vi "__Local List Menu Delete Handler.vi"(7 "FileManager Data":T1, 8 "error in (no error)":errorcluster) -> (0 "error out":errorcluster)   [LabVIEW 2011]
doc: "Handles the delete operation on the Local list."
uses:
  __File manager Data type.ctl
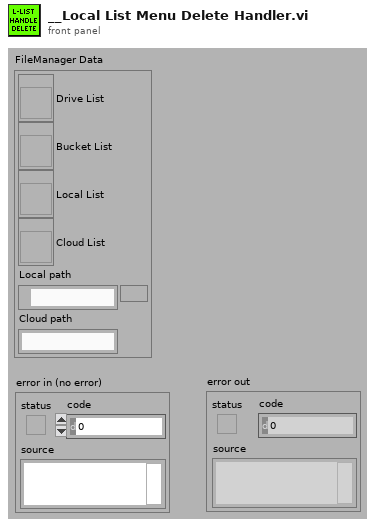
[diagram p1: front panel]
types:
  T1 = typedef "__File manager Data type.ctl" = cluster{"Drive List":refnum<vi>, "Bucket List":refnum<vi>, "Local List":refnum<vi>, "Cloud List":refnum<vi>, "Local path":path, "Cloud path":string}
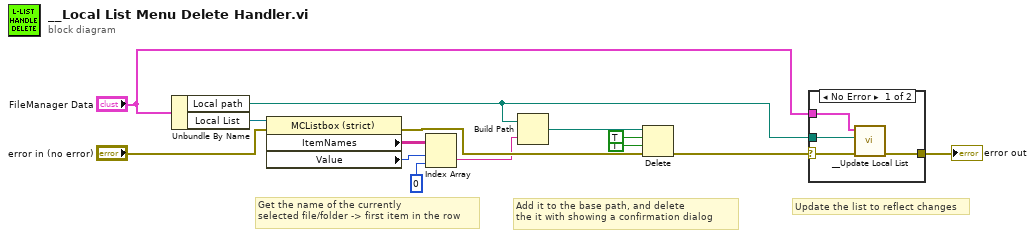
[diagram p0: block diagram]
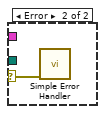
[diagram p2: hidden frame]
diagram:
  # "Update the list to reflect changes"
  # "Add it to the base path, and delete\nthe it with showing a confirmation dialog"
  # "Get the name of the currently\nselected file/folder -> first item in the row"
  n1 = Unbundle By Name("FileManager Data") -> ("Local path"=w3:path, "Local List"=w6:refnum<vi>)
  n2 = property class="MCListbox (strict)"(reference=w6, error in="error in (no error)") -> (error out=w4:errorcluster, "ItemNames"=w9:string[][], "Value"=w8:i32)  [unwired: 1 out]
  n3 = Index Array(array=w9, index (row)=w8, index (col)=0 ("disabled index (col)")) -> (element=w2:string)
  n4 = Build Path(base path=w3, name or relative path=w2) -> (appended path=w1:path)
  n5 = Delete(path (use dialog)=w1, entire hierarchy (F)=TRUE, confirm (F)=TRUE, error in=w4) -> (error out=w10:errorcluster)  [unwired: 1 in, 2 out]
  n6 = case shown="No Error" w10 {
    selector: w10 -> [w18 w19]
    tunnel: [w17 _] -> w14
    tunnel: "FileManager Data" -> [w15 _]
    tunnel: w3 -> [w16 _]
    frame No Error {
      n7 = call "__Update Local List.vi"("error in (no error)"=w18, "Path to list"=w16, "FileManager Ctl Refs in"=w15) -> ("error out"=w17:errorcluster)  [unwired: 7 in, 1 out]
    }
    frame Error {
      n8 = call <vilib>:"Simple Error Handler.vi"("error in (no error)"=w19) -> ()  [unwired: 4 in, 5 out]
    }
  }
  "error out" <- w14
